vi "Check Dependencies.vi"(10 "Variant":variant) -> (0 "error out":errorcluster)   [LabVIEW 2011]
uses:
  <vilib>/LabVIEW Hacker/LVH-Toolbox/Installer Tools/Installer Tools.lvlib
  <vilib>/LabVIEW Hacker/LVH-Toolbox/Common/LVH-Common.lvlib
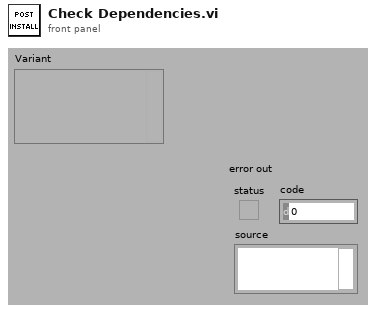
[diagram p1: front panel]
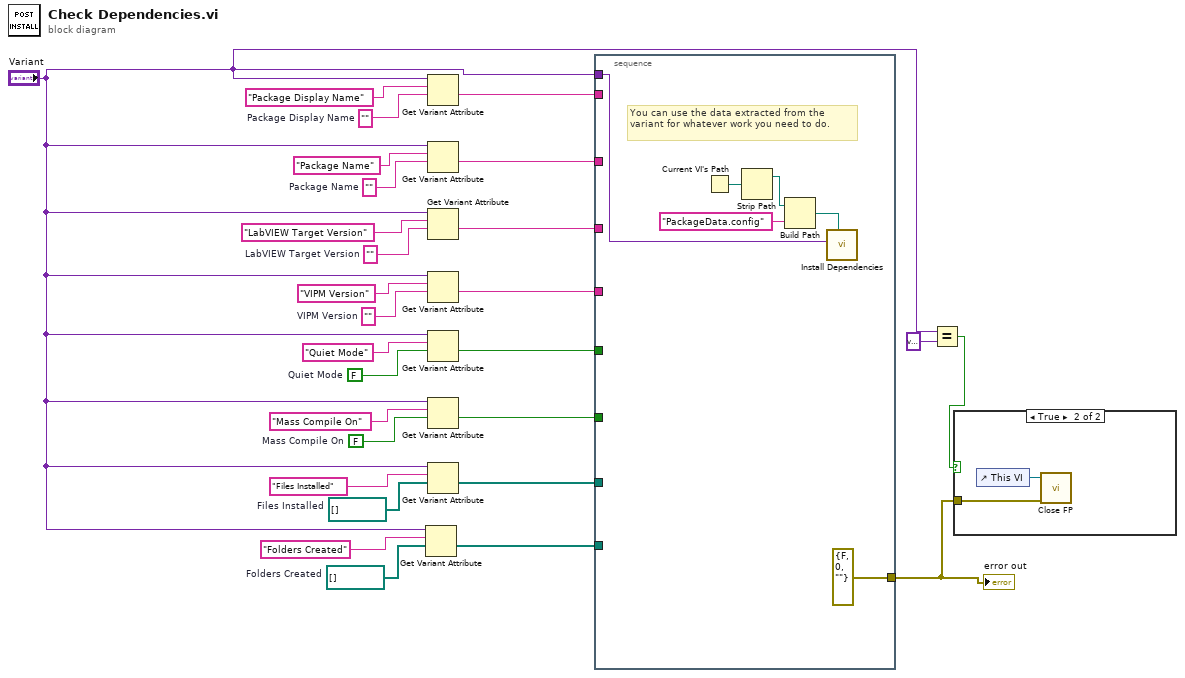
[diagram p0: block diagram]
diagram:
  w5 = path[] []  # Folders Created
  w6 = path[] []  # Files Installed
  w11 = FALSE  # Mass Compile On
  w12 = ""  # Package Display Name
  w19 = FALSE  # Quiet Mode
  w22 = ""  # VIPM Version
  w24 = ""  # LabVIEW Target Version
  w26 = ""  # Package Name
  n1 = Get Variant Attribute(Variant="Variant", name="Folders Created", default value (empty Variant)=w5) -> (value=w9:path[])  [unwired: 1 in, 3 out]
  n2 = Get Variant Attribute(Variant="Variant", name="Package Display Name", default value (empty Variant)=w12) -> (value=w18:string)  [unwired: 1 in, 3 out]
  n3 = Get Variant Attribute(Variant="Variant", name="Package Name", default value (empty Variant)=w26) -> (value=w17:string)  [unwired: 1 in, 3 out]
  n4 = Get Variant Attribute(Variant="Variant", name="LabVIEW Target Version", default value (empty Variant)=w24) -> (value=w16:string)  [unwired: 1 in, 3 out]
  n5 = Get Variant Attribute(Variant="Variant", name="VIPM Version", default value (empty Variant)=w22) -> (value=w15:string)  [unwired: 1 in, 3 out]
  n6 = Get Variant Attribute(Variant="Variant", name="Quiet Mode", default value (empty Variant)=w19) -> (value=w14:bool)  [unwired: 1 in, 3 out]
  n7 = Get Variant Attribute(Variant="Variant", name="Mass Compile On", default value (empty Variant)=w11) -> (value=w13:bool)  [unwired: 1 in, 3 out]
  n8 = Get Variant Attribute(Variant="Variant", name="Files Installed", default value (empty Variant)=w6) -> (value=w8:path[])  [unwired: 1 in, 3 out]
  n9 = stacked-sequence {
    tunnel: w18 -> [_]
    tunnel: w17 -> [_]
    tunnel: w16 -> [_]
    tunnel: w15 -> [_]
    tunnel: w14 -> [_]
    tunnel: w13 -> [_]
    tunnel: w8 -> [_]
    tunnel: w9 -> [_]
    tunnel: [errorcluster {"status"=FALSE, "code"=0, "source"=""} ("error out")] -> w4
    tunnel: "Variant" -> [w29]
    frame #0 {
      # "You can use the data extracted from the variant for whatever work you need to do."
      n10 = Current VI's Path() -> (path=w31:path)
      n11 = Strip Path(path=w31) -> (stripped path=w32:path)  [unwired: 1 out]
      n12 = Build Path(base path=w32, name or relative path="PackageData.config") -> (appended path=w34:path)
      n13 = call <vilib>:"Install Dependencies.vi"("Stored Install Data"=w34, "Variant"=w29) -> ()  [unwired: 9 in, 1 out]
    }
  }
  "error out" <- w4
  n14 = Equal?(x="Variant", y=variant) -> (x = y?=w1:bool)
  n15 = case shown="True" w1 {
    tunnel: w4 -> [_ w35]
    frame False {
    }
    frame True {
      n16 = control-ref of="This VI"() -> (w36:refnum<vi>)
      n17 = call <vilib>:"Close FP.vi"("Error In"=w35, "VI Ref"=w36) -> ()  [unwired: 9 in, 1 out]
    }
  }
